vi "TL Motor MoveComplete CallBack.vi"(4 "User Parameter":variant, 5 "Event Data":cluster{"lChanID":i32}, 6 "Control Ref":refnum<k7>, 7 "Event Common Data":T1) -> ()   [LabVIEW 2021]
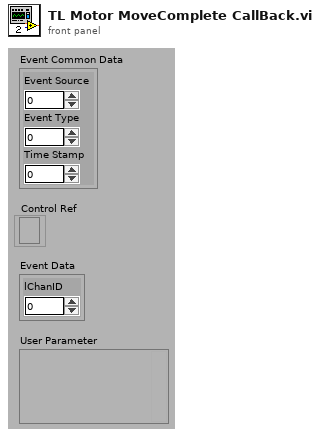
[diagram p1: front panel]
types:
  T1 = cluster{"Event Source":i32, "Event Type":u32, "Time Stamp":u32}
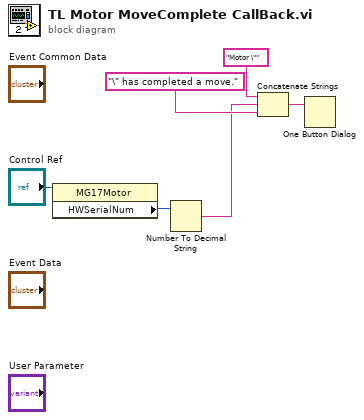
[diagram p0: block diagram]
diagram:
  n1 = property class="MG17Motor"(reference="Control Ref") -> ("HWSerialNum"=w3:i32)  [unwired: 1 in, 2 out]
  n2 = Number To Decimal String(number=w3) -> (decimal integer string=w2:string)  [unwired: 1 in]
  n3 = Concatenate Strings("Motor \"" ("string"), w2, "\" has completed a move." ("string")) -> (w1:string)
  n4 = One Button Dialog(message=w1) -> ()  [unwired: 1 in, 1 out]
